vi "reporteexcel.vi"() -> ()   [LabVIEW 2016]
uses:
  <vilib>/addons/_office/_exclsub.llb/font.ctl
  <vilib>/addons/_office/excel.llb/Excel Easy Table (num).vi
  <vilib>/printing/ReportDocExtensions.llb/Append Front Panel Image to Report (path).vi
  <vilib>/printing/ReportDocExtensions.llb/Append VI Block Diagram to Report (path).vi
  <vilib>/Utility/NIReport.llb/NI_report.lvclass
  <vilib>/addons/_office/NI_ReportGenerationToolkit.lvlib
  <vilib>/Utility/NIReport.llb/NI_ReportGenerationCore.lvlib
panel:
  out "start (0, 0)":cluster{"row":i32, "column":i32}
  in  "report file path":path=path "C:/Users/Silvia/Desktop/tareas/instrumentacion virtual/exc"
  in  "VI":path
  out "Gauge":dbl(knob) scale=0.0..10.0
  out "XY Graph":cluster{"X":dbl, "Y":dbl}[](graph)
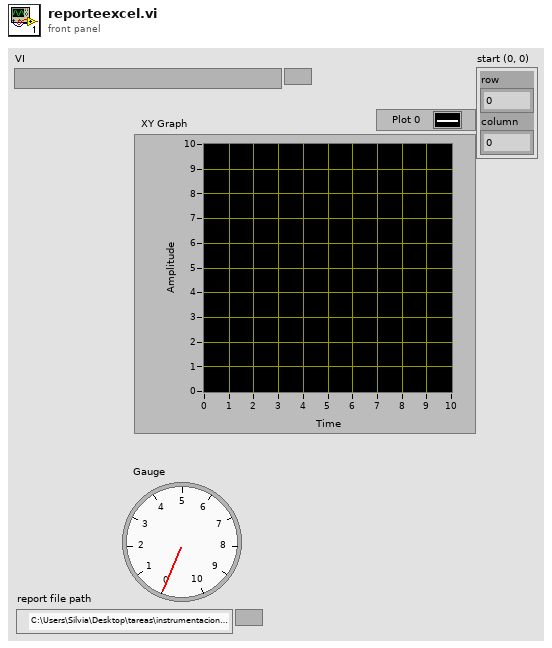
[diagram p1: front panel]
types:
  T1 = cluster{"position (Excel)":cluster{"row":i32, "column":i32}, "name (Excel)":string, "bookmark (Word)":string}
  T2 = typedef "NI_ReportGenerationToolkit.lvlib/font.ctl" = cluster{"font name":string, "font size":dbl, "bold":u16, "italic":u16, "underline":u16, "strike through":u16, "font color":u32}
  T3 = enum16{"xlColumnClustered", "xlColumnStacked", "xlColumnStacked100", "xl3DColumnClustered", "xl3DColumnStacked", "xl3DColumnStacked100", "xlBarClustered", "xlBarStacked", "xlBarStacked100", "xl3DBarClustered", "xl3DBarStacked", "xl3DBarStacked100", "xlLineStacked", "xlLineStacked100", "xlLineMarkers", "xlLineMarkersStacked", "xlLineMarkersStacked100", "xlPieOfPie", "xlPieExploded", "xl3DPieExploded", "xlBarOfPie", "xlXYScatterSmooth", "xlXYScatterSmoothNoMarkers", "xlXYScatterLines", "xlXYScatterLinesNoMarkers", "xlAreaStacked", "xlAreaStacked100", "xl3DAreaStacked", "xl3DAreaStacked100", "xlDoughnutExploded", "xlRadarMarkers", "xlRadarFilled", "xlSurface", "xlSurfaceWireframe", "xlSurfaceTopView", "xlSurfaceTopViewWireframe", "xlBubble", "xlBubble3DEffect", "xlStockHLC", "xlStockOHLC", "xlStockVHLC", "xlStockVOHLC", "xlCylinderColClustered", "xlCylinderColStacked", "xlCylinderColStacked100", "xlCylinderBarClustered", "xlCylinderBarStacked", "xlCylinderBarStacked100", "xlCylinderCol", "xlConeColClustered", "xlConeColStacked", "xlConeColStacked100", "xlConeBarClustered", "xlConeBarStacked", "xlConeBarStacked100", "xlConeCol", "xlPyramidColClustered", "xlPyramidColStacked", "xlPyramidColStacked100", "xlPyramidBarClustered", "xlPyramidBarStacked", "xlPyramidBarStacked100", "xlPyramidCol", "xl3DColumn", "xlLine", "xl3DLine", "xl3DPie", "xlPie", "xlXYScatter", "xl3DArea", "xlArea", "xlDoughnut", "xlRadar"}
  T4 = enum16{"Standard Report", "HTML", "Word", "Excel"}
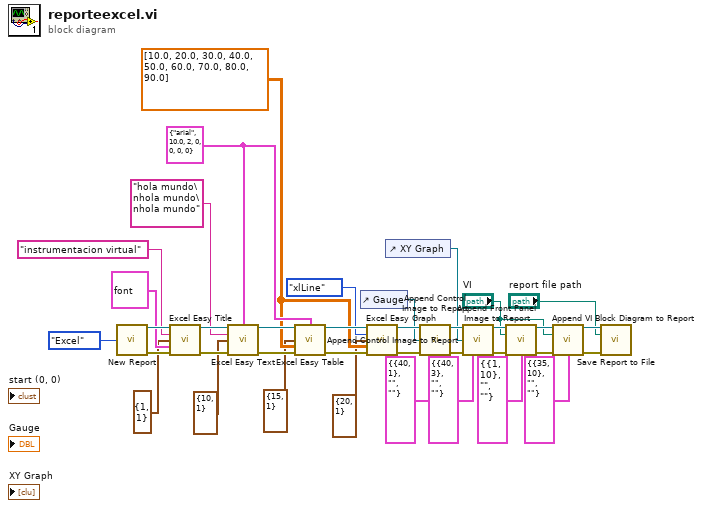
[diagram p0: block diagram]
diagram:
  w24 = T2 {"font name"="arial", "font size"=10.0, "bold"=2, "italic"=0, "underline"=0, "strike through"=0, "font color"=0} ("font")
  w9 = dbl[][] [[10.0, 20.0, 30.0], [40.0, 50.0, 60.0], [70.0, 80.0, 90.0]] ("text data")
  n1 = call <vilib>:"New Report.vi"("report type"=T4."Excel") -> ("report out"=w36:refnum<class "NI_report.lvclass">, "error out"=w35:errorcluster)  [unwired: 13 in]
  n2 = call <vilib>:"Excel Easy Title.vi"("report in"=w36, "title"="instrumentacion virtual", "start (0, 0)"=cluster{"row":i32, "column":i32} {"row"=1, "column"=1}, "font"=T2 {"font name"="impact", "font size"=36.0, "bold"=1, "italic"=0, "underline"=0, "strike through"=0, "font color"=16716306}, "error in (no error)"=w35) -> ("report out"=w33:refnum<class "NI_report.lvclass">, "error out"=w32:errorcluster)  [unwired: 8 in, 1 out]
  n3 = call <vilib>:"Excel Easy Text.vi"("report in"=w33, "font"=w24, "text"="hola mundo\nhola mundo\nhola mundo", "start (-1, -1)"=cluster{"row":i32, "column":i32} {"row"=10, "column"=1}, "error in (no error)"=w32) -> ("report out"=w30:refnum<class "NI_report.lvclass">, "error out"=w29:errorcluster)  [unwired: 6 in, 3 out]
  n4 = call-poly <vilib>:"Excel Easy Table.vi"("report in"=w30, "font"=w24, "start (0, 0)"=cluster{"row":i32, "column":i32} {"row"=15, "column"=1}, "text data"=w9, "error in (no error)"=w29) -> ("report out"=w28:refnum<class "NI_report.lvclass">, "error out"=w27:errorcluster)  [unwired: 6 in, 3 out]
  n5 = control-ref of="Gauge"() -> (w19:refnum<vi>)
  n6 = call <vilib>:"Excel Easy Graph.vi"("report in"=w28, "graph type (col clustered)"=T3."xlLine", "start (0, 0)"=cluster{"row":i32, "column":i32} {"row"=20, "column"=1}, "data"=w9, "error in (no error)"=w27) -> ("report out"=w23:refnum<class "NI_report.lvclass">, "error out"=w22:errorcluster)  [unwired: 9 in]
  n7 = control-ref of="XY Graph"() -> (w18:refnum<vi>)
  n8 = call-dynamic "Append Control Image to Report.vi"("report in"=w23, "ctrl reference"=w19, "error in (no error)"=w22, "MS Office parameters"=T1 {"position (Excel)"={"row"=40, "column"=1}, "name (Excel)"="", "bookmark (Word)"=""}) -> ("report out"=w21:refnum<class "NI_report.lvclass">, "error out"=w20:errorcluster)  [unwired: 8 in, 2 out]
  n9 = call-dynamic "Append Control Image to Report.vi"("report in"=w21, "ctrl reference"=w18, "error in (no error)"=w20, "MS Office parameters"=T1 {"position (Excel)"={"row"=40, "column"=3}, "name (Excel)"="", "bookmark (Word)"=""}) -> ("report out"=w17:refnum<class "NI_report.lvclass">, "error out"=w16:errorcluster)  [unwired: 8 in, 2 out]
  n10 = call-poly <vilib>:"Append Front Panel Image to Report.vi"("report in"=w17, "VI"="VI", "error in (no error)"=w16, "MS Office parameters"=T1 {"position (Excel)"={"row"=1, "column"=10}, "name (Excel)"="", "bookmark (Word)"=""}) -> ("report out"=w15:refnum<class "NI_report.lvclass">, "error out"=w14:errorcluster)  [unwired: 7 in, 3 out]
  n11 = call-poly <vilib>:"Append VI Block Diagram to Report.vi"("report in"=w15, "VI"="VI", "error in (no error)"=w14, "MS Office parameters"=T1 {"position (Excel)"={"row"=35, "column"=10}, "name (Excel)"="", "bookmark (Word)"=""}) -> ("report out"=w12:refnum<class "NI_report.lvclass">, "error out"=w11:errorcluster)  [unwired: 7 in, 3 out]
  n12 = call-dynamic "Save Report to File.vi"("report in"=w12, "report file path"="report file path", "error in (no error)"=w11) -> ()  [unwired: 11 in, 2 out]
